vi "Introspection Core.vi"(8 "error in (no error)":errorcluster, 11 "PVClient-Example in":refnum<class "PVClient-Example.lvclass">) -> (0 "error out":errorcluster, 2 "CS++Messages":refnum<class "Message.lvclass">[](array[class]), 3 "PVClient-Example out":refnum<class "PVClient-Example.lvclass">)   [LabVIEW 2016, in "PVClient-Example.lvlib" / "PVClient-Example.lvclass"]
doc: "This vi delivers a list with all messages this actor reacts to. \n\nNote that all inherited classes have to overwrite it."
uses:
  PVClient-Example.lvclass
  <vilib>/ActorFramework/Message/Message.lvclass
  PVClient-Example Messages/AEUpdate Msg/AEUpdate Msg.lvclass
  C:/Program Files (x86)/National Instruments/LabVIEW 2016/vi.lib/ActorFramework/Message/Message.lvclass
  PVClient-Example Messages/PVUpdate-myDouble Msg/PVUpdate-myDouble Msg.lvclass
  CSPP_Core/Actors/CS++BaseActor/CS++BaseActor.lvclass
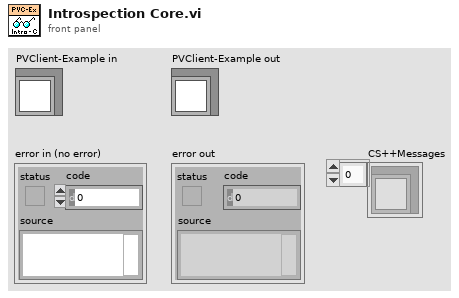
[diagram p1: front panel]
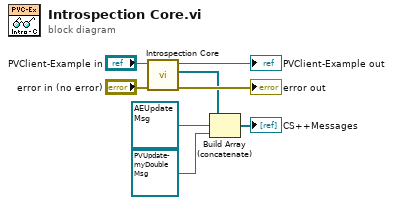
[diagram p0: block diagram]
diagram:
  n1 = call-parent "Introspection Core.vi"("error in (no error)"="error in (no error)", "CS++BaseActor in"="PVClient-Example in") -> ("error out"=→"error out":errorcluster, "CS++Messages"=w7:refnum<class "Message.lvclass">[], "CS++BaseActor out"=→"PVClient-Example out":refnum<class "PVClient-Example.lvclass">)  [unwired: 7 in]
  n2 = Build Array (concatenate)(w7, refnum<class "AEUpdate Msg.lvclass"> refnum ("PVClient-Example.lvlib:AEUpdate Msg.lvclass"), refnum<class "PVUpdate-myDouble Msg.lvclass"> refnum ("PVClient-Example.lvlib:PVUpdate-myDouble Msg.lvclass")) -> (→"CS++Messages":refnum<class "Message.lvclass">[])
